vi "Update proto text.vi"(8 "error in":errorcluster, 10 "New Subname":string, 11 "Proto Text In":string) -> (0 "error out":errorcluster, 2 "Proto Names":T1={"PascalCase"="Plugin8", "snake_case"="plugin_8"}, 3 "Proto Text Out":string)   [LabVIEW 2021, in "Plugin Generator.lvlib"]
uses:
  Plugin Generator.lvlib
  Typedef/Proto Names.ctl
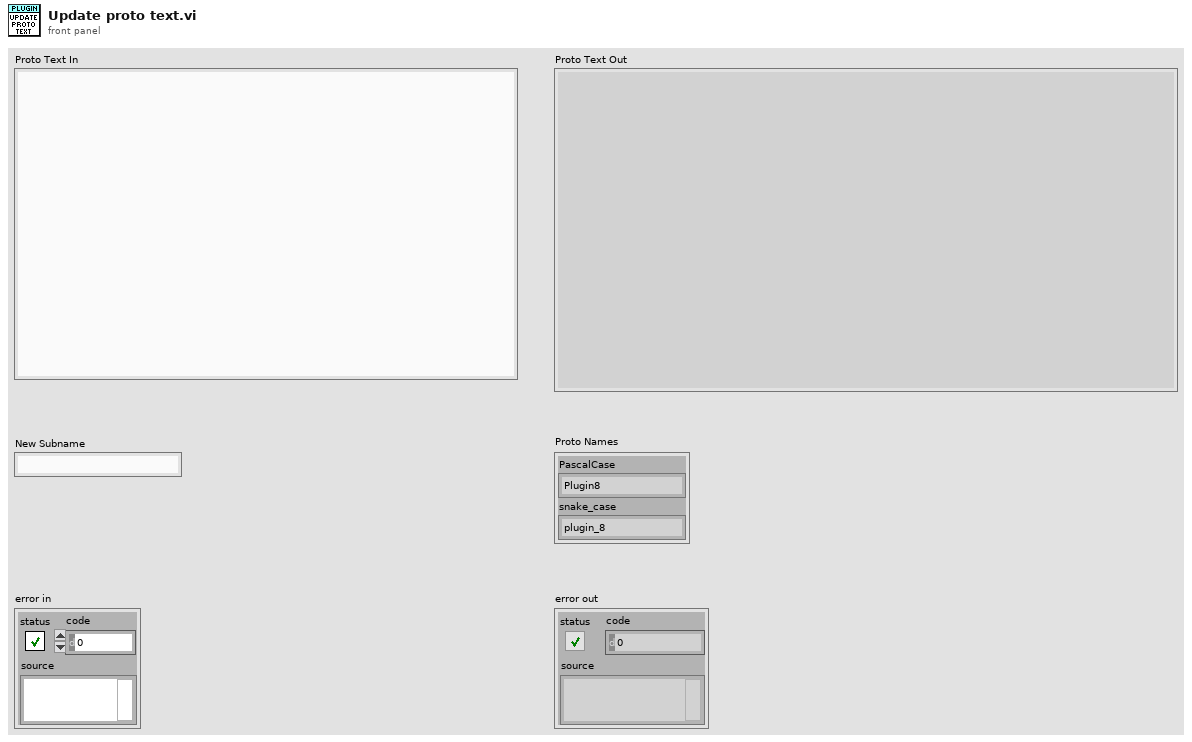
[diagram p1: front panel]
types:
  T1 = typedef "Plugin Generator.lvlib/Proto Names.ctl" = cluster{"PascalCase":string, "snake_case":string}
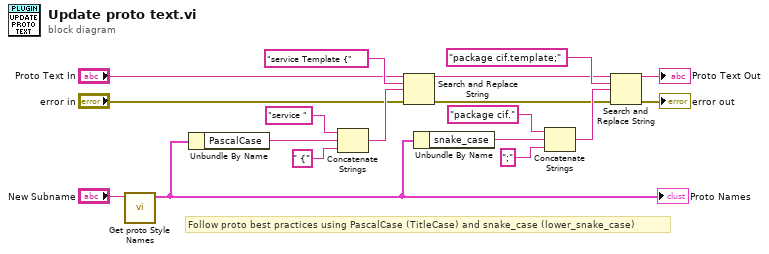
[diagram p0: block diagram]
diagram:
  # "Follow proto best practices using PascalCase (TitleCase) and snake_case (lower_snake_case)"
  n1 = call "Get proto Style Names.vi"("Input Name"="New Subname") -> ("Proto Names"=w2:T1)  [unwired: 10 in]
  "Proto Names" <- w2
  n2 = Unbundle By Name(w2) -> ("PascalCase"=w3:string)
  n3 = Concatenate Strings("service ", w3, " {") -> (w17:string)
  n4 = Search and Replace String(input string="Proto Text In", search string="service Template {", replace string=w17, error in="error in") -> (result string=w7:string, error out=w6:errorcluster)  [unwired: 4 in, 2 out]
  n5 = Unbundle By Name(w2) -> ("snake_case"=w1:string)
  n6 = Concatenate Strings("package cif.", w1, ";") -> (w8:string)
  n7 = Search and Replace String(input string=w7, search string="package cif.template;", replace string=w8, error in=w6) -> (result string=→"Proto Text Out":string, error out=→"error out":errorcluster)  [unwired: 4 in, 2 out]
